vi "Circulo.vi"(0 "Radio":dbl) -> (1 "Area":dbl, 2 "Perimetro":dbl)   [LabVIEW 2016]
doc: "Este VI se dedica a obtener el area y el perimetro de un circulo dando el radio como entrada"
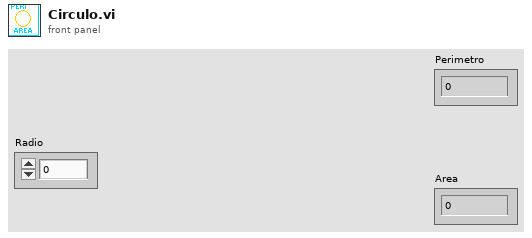
[diagram p1: front panel]
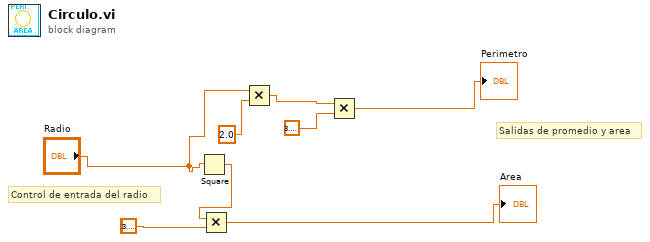
[diagram p0: block diagram]
diagram:
  (unwired) 3.141592653589793
  # "Salidas de promedio y area"
  # "Control de entrada del radio"
  n1 = Square(x="Radio") -> (x^2=w2:dbl)
  n2 = Multiply(x=w2, y=3.141592653589793) -> (x*y=→"Area":dbl)
  n3 = Multiply(x="Radio", y=2.0) -> (x*y=w6:dbl)
  n4 = Multiply(x=w6, y=3.141592653589793) -> (x*y=→"Perimetro":dbl)
